vi "CRYPreload Operator Window.vi"   [LabVIEW 2013]
uses:
  SubVI/CRYMisc vis settings global.vi
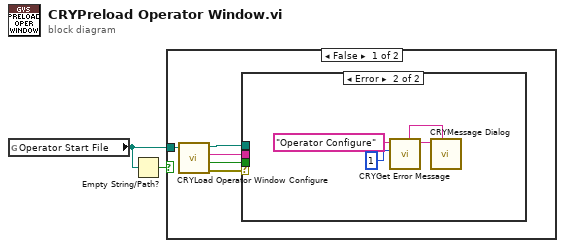
[diagram p0: block diagram]
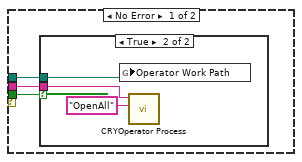
[diagram p2: hidden frame]
diagram:
  n1 = global read "CRYMisc vis settings global.vi" "Operator Start File"() -> (w2:path)
  n2 = Empty String/Path?(string/path=w2) -> (empty?=w1:bool)
  n3 = case shown="False" w1 {
    tunnel: w2 -> [w3 _]
    frame False {
      n4 = call "CRYLoad Operator Window Configure.vi"("File path"=w3) -> ("error out"=w4:errorcluster, "ok status"=w6:bool, "Flatten Step"=w7:string, "selected path"=w5:path)  [unwired: 7 in]
      n5 = case shown="Error" w4 {
        tunnel: w7 -> [w9 _]
        tunnel: w6 -> [w10 _]
        tunnel: w5 -> [w8 _]
        frame No Error {
          n6 = case shown="True" w10 {
            tunnel: w9 -> [_ w13]
            tunnel: w8 -> [_ w12]
            frame False {
            }
            frame True {
              n7 = global write "CRYMisc vis settings global.vi" "Operator Work Path"(w12) -> ()
              n8 = call "CRYOperator Process.vi"("sAction"="OpenAll", "sOperator Type"=w13) -> ()  [unwired: 9 in, 1 out]
            }
          }
        }
        frame Error {
          n9 = call "CRYGet Error Message.vi"("Error No"=1, "Kind"="Operator Configure") -> ("Message"=w17:string, "Window Title"=w16:string)  [unwired: 4 in, 4 out]
          n10 = call "CRYMessage Dialog.vi"("Window Title"=w16, "Message Content"=w17) -> ()  [unwired: 8 in, 2 out]
        }
      }
    }
    frame True {
    }
  }
